vi "Read Attributes.vi"(11 "Return DeviceID Array Msg":refnum<class "Return DeviceID Array Msg.lvclass">) -> (2 "Payload":cluster{"DeviceID Array":T1[]})   [LabVIEW 2018, in "EMS Core.lvlib" / "Return DeviceID Array Msg.lvclass"]
uses:
  Return DeviceID Array Msg.lvclass
  <vilib>/ORNL/CSEISMIC DDS/CSEISMIC DDS Base/Data Types/Controls/DeviceID.ctl
  Return DeviceID Array Msg.lvclass/Return DeviceID Array Msg.ctl
  <vilib>/ORNL/CSEISMIC DDS/CSEISMIC DDS Base/CSEISMIC DDS.lvclass
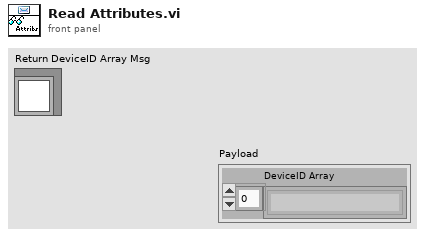
[diagram p1: front panel]
types:
  T1 = typedef "CSEISMIC DDS.lvlib/CSEISMIC DDS.lvclass/DeviceID.ctl" = string
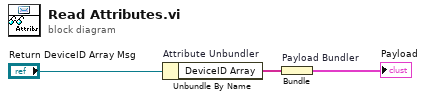
[diagram p0: block diagram]
diagram:
  n1 = Unbundle By Name "Attribute Unbundler"("Return DeviceID Array Msg") -> ("DeviceID Array"=w1:T1[])
  n2 = Bundle "Payload Bundler"("DeviceID Array"=w1) -> (→"Payload":cluster{"DeviceID Array":T1[]})  [unwired: 1 in]
